vi "DB UI - MasterData SAPProduction Long Text.vi"(7 "DB Connection":T3={"Open"=TRUE, "Close"=TRUE}, 8 "error in (no error)":errorcluster, 9 "[OrderNo]":string, 10 "[PlantId]":string, 11 "connection reference 2":T1) -> (0 "SUMMARY":errorcluster, 3 "connection reference":T1)   [LabVIEW 2013]
uses:
  <vilib>/addons/database/Connection.llb/Conn ObjectReference.ctl
  Controls/DB - OpenClose.ctl
  <vilib>/Utility/miscctls.llb/LVPointTypeDef.ctl
  Controls/Global SRTRS.vi
  <vilib>/addons/database/Connection.llb/DB Tools Open Connec (String).vi
  <vilib>/addons/database/NI_Database_API.lvlib
panel:
  in  "Tab Control":enum32{"Debug"}(tab)
  out "Connection Information":T2={"Connection "="SQL Server 32bit HPEnvy", "Username"="admin", "Password"="admin123"}
  in  "SRTRS.MasterData.SAPProduction":string="SRTRS.MasterData.SAPProduction"
  out "SQL Statement":string
  out "Close 2":errorcluster
  out "[LongText]":string caption="Long Text"
  in  "Close":bool caption="Setup Save"
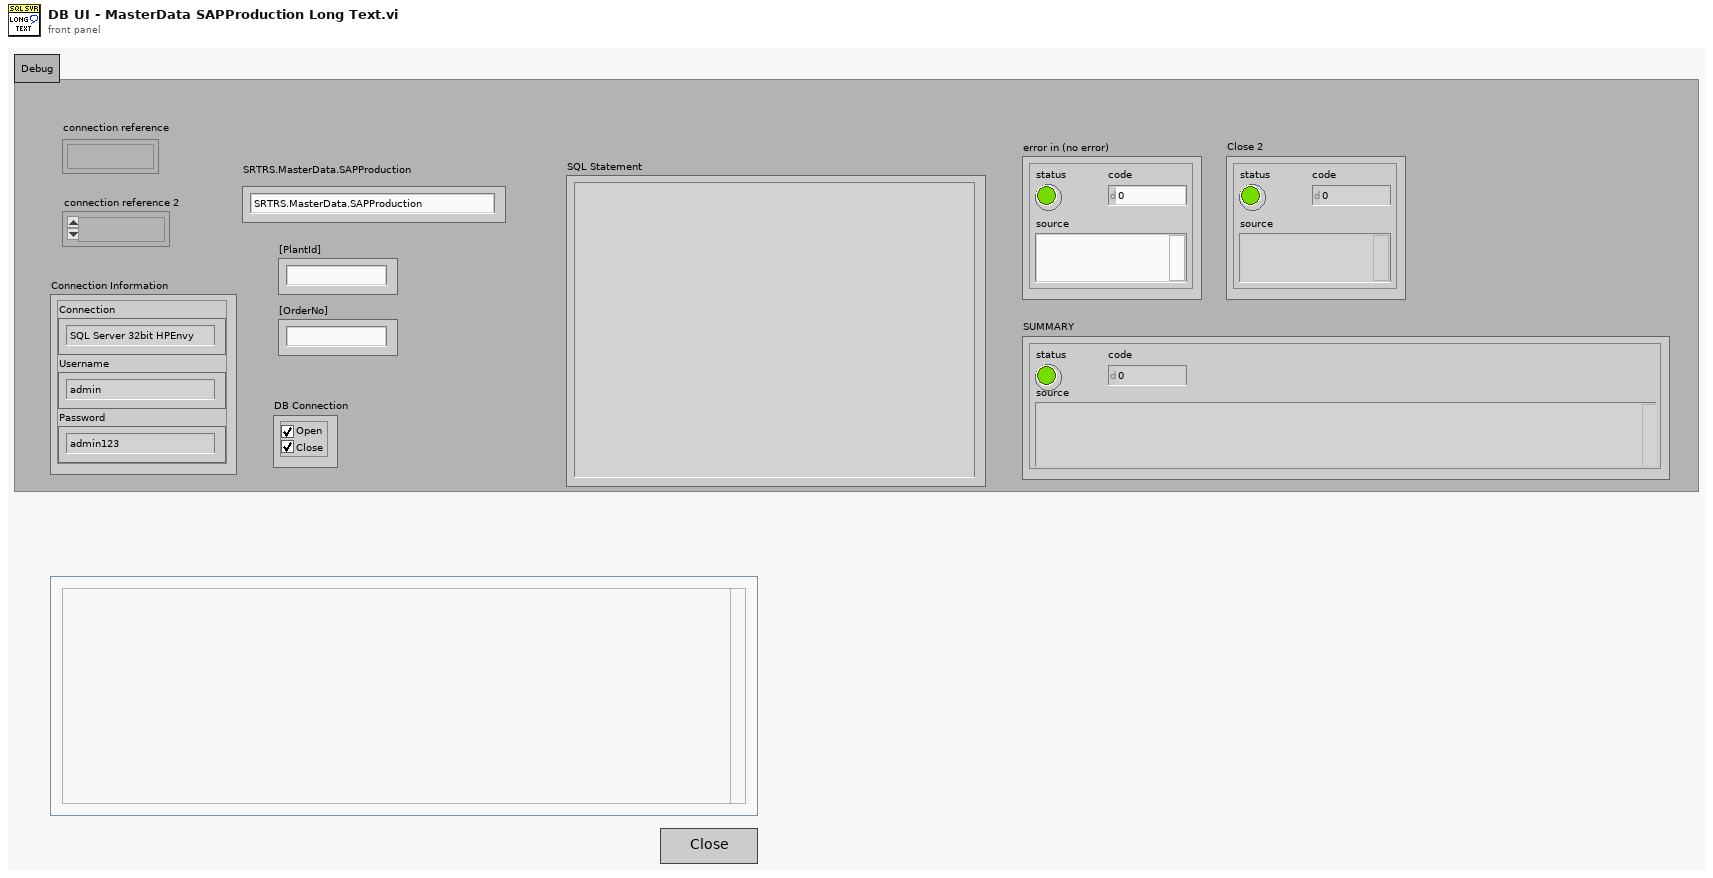
[diagram p1: front panel]
types:
  T1 = typedef "NI_Database_API.lvlib/Conn ObjectReference.ctl" = refnum<k1>
  T2 = cluster{"Connection ":string, "Username":string, "Password":string}
  T3 = typedef "DB - OpenClose.ctl" = cluster{"Open":bool, "Close":bool}
  T4 = typedef "LVPointTypeDef.ctl" = cluster{"Horizontal":i16, "Vertical":i16}
  T5 = typedef "Enum - InteractiveMode-SubVIMode.ctl" = enum16{"Interactive", "subVI Mode"}
  T6 = typedef "DB - DB.Schema.Table.ctl" = cluster{"DB":string, "Schema":string, "Table":string}
  T7 = typedef "Connection Information Cluster.ctl" = cluster{"Connection ":string, "Username":string, "Password":string}
  T8 = typedef "DB - Logon Extra Info.ctl" = cluster{"Plant Name":string, "UserName":string, "Hostname [ClientName]":string, "IsUnicode":bool}
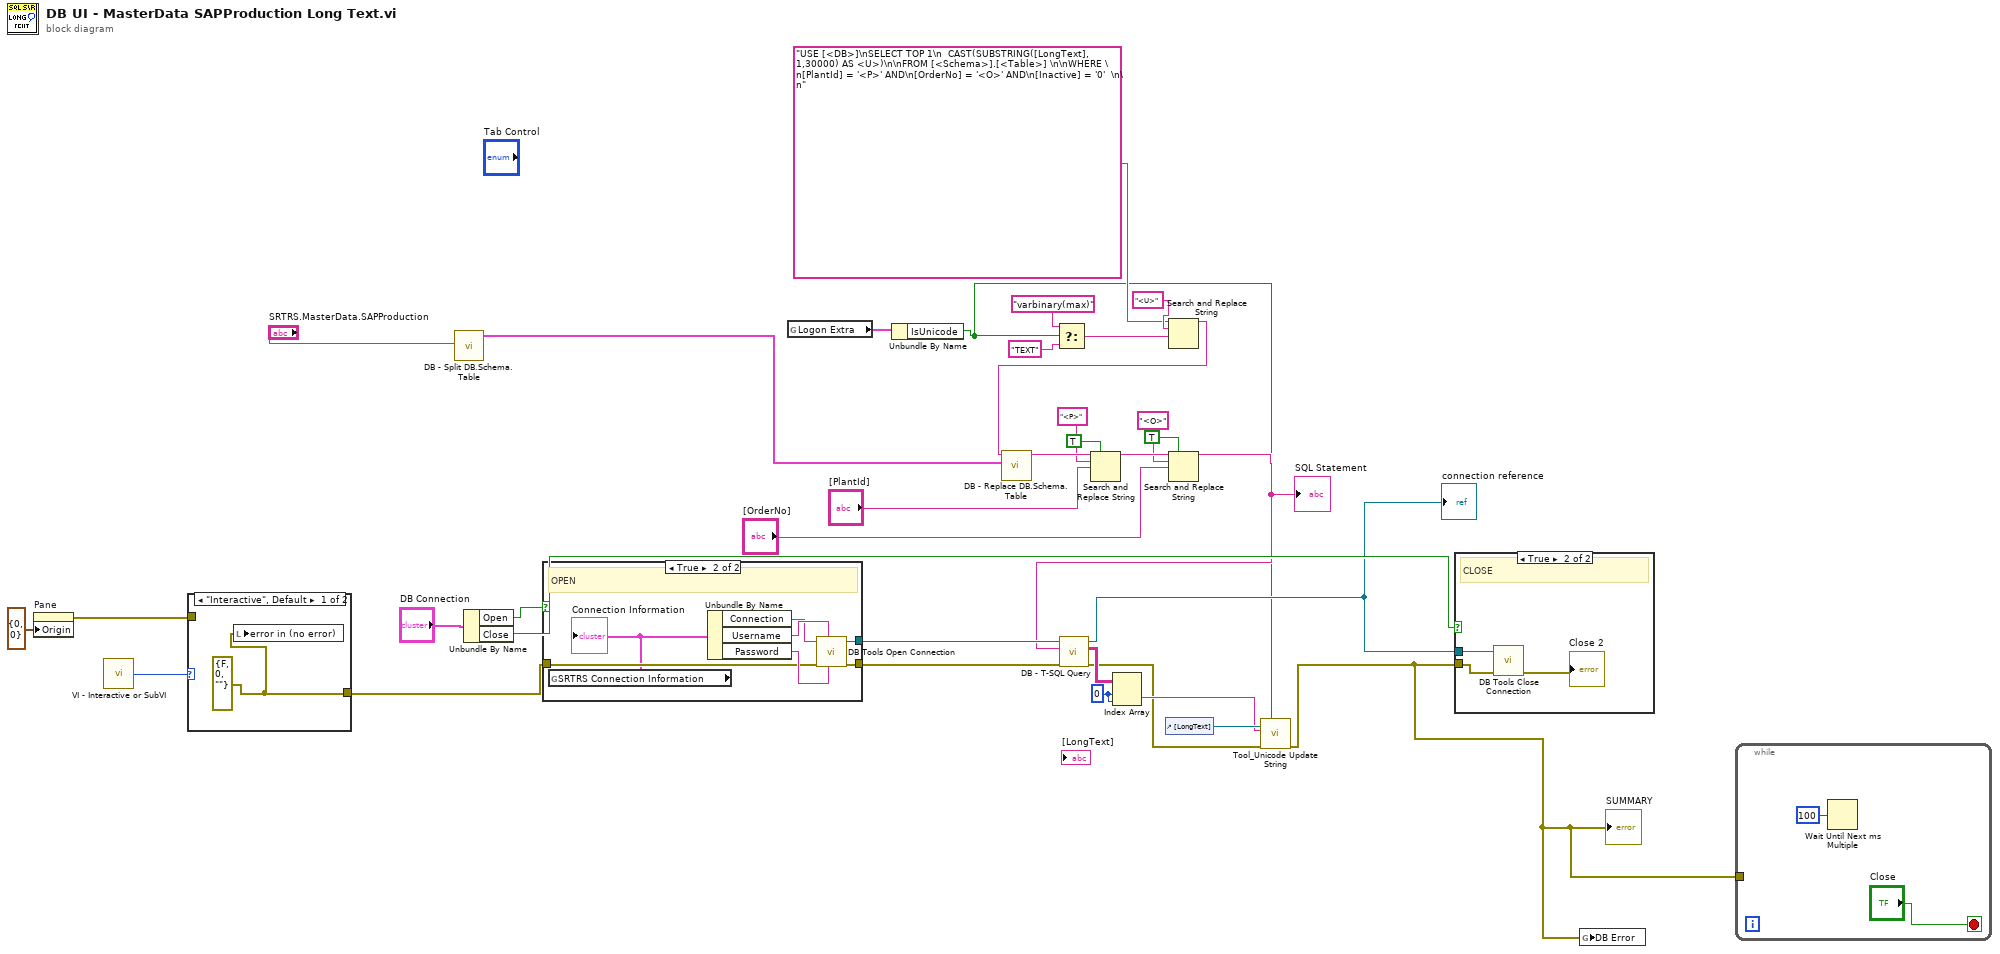
[diagram p0: block diagram]
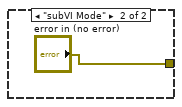
[diagram p3: hidden frame]
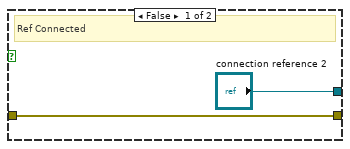
[diagram p4: hidden frame]
diagram:
  w20 = 0 ("index (row)")
  n1 = property on="Pane" class="Pane"("Origin"=T4 {"Horizontal"=0, "Vertical"=0}) -> (error out=w24:errorcluster)  [unwired: 2 in, 1 out]
  n2 = call "VI - Interactive or SubVI.vi"() -> ("Mode"=w33:T5)  [unwired: 5 in]
  n3 = case shown="\"Interactive\", Default" w33 {
    tunnel: [w36 "error in (no error)"] -> w32
    tunnel: w24 -> [_ _]
    frame "Interactive", Default {
      w36 = errorcluster {"status"=FALSE, "code"=0, "source"=""} ("error in (no error)")
      n4 = local write "error in (no error)"(w36) -> ()
    }
    frame "subVI Mode" {
    }
  }
  n5 = call "DB - Split DB.Schema.Table.vi"("DB.Schema.Table"="SRTRS.MasterData.SAPProduction") -> ("DB.Schema.Table"=w29:T6)  [unwired: 10 in]
  n6 = Unbundle By Name("DB Connection") -> ("Open"=w34:bool, "Close"=w31:bool)
  n7 = case shown="True" w34 {
    tunnel: ["connection reference 2" w43] -> w23
    tunnel: w32 -> [w38 w42]
    tunnel: [w38 w41] -> w22
    frame False {
      # "Ref Connected"
    }
    frame True {
      # "OPEN"
      n8 = global read "Global SRTRS.vi" "SRTRS Connection Information"() -> (w40:T7)
      "Connection Information" <- w40
      n9 = Unbundle By Name(w40) -> ("Connection"=w45:string, "Username"=w46:string, "Password"=w44:string)
      n10 = call-poly <vilib>:"DB Tools Open Connection.vi"("password"=w44, "userID"=w46, "error in (no error)"=w42, "connection information"=w45) -> ("error out"=w41:errorcluster, "connection reference"=w43:T1)  [unwired: 4 in]
    }
  }
  n11 = global read "Global SRTRS.vi" "Logon Extra"() -> (w6:T8)
  n12 = Unbundle By Name(w6) -> ("IsUnicode"=w5:bool)
  n13 = Select(t="varbinary(max)", s=w5, f="TEXT") -> (s? t:f=w11:string)
  n14 = control-ref of="[LongText]"() -> (w4:refnum<vi>)
  n15 = Search and Replace String(input string="USE [<DB>]\nSELECT TOP 1\n  CAST(SUBSTRING([LongText], 1,30000) AS <U>)\n\nFROM [<Schema>].[<Table>] \n\nWHERE \n[PlantId] = '<P>' AND\n[OrderNo] = '<O>' AND\n[Inactive] = '0'  \n\n", search string="<U>", replace string=w11) -> (result string=w7:string)  [unwired: 5 in, 3 out]
  n16 = call "DB - Replace DB.Schema.Table.vi"("DB.Schema.Table"=w29, "string in"=w7) -> ("string out"=w28:string)  [unwired: 8 in, 1 out]
  n17 = Search and Replace String(replace all?=TRUE ("replace all? (F)"), input string=w28, search string="<P>", replace string="[PlantId]") -> (result string=w18:string)  [unwired: 4 in, 3 out]
  n18 = Search and Replace String(replace all?=TRUE ("replace all? (F)"), input string=w18, search string="<O>", replace string="[OrderNo]") -> (result string=w17:string)  [unwired: 4 in, 3 out]
  "SQL Statement" <- w17
  n19 = call "DB - T-SQL Query.vi"("error in (no error)"=w22, "T-SQL"=w17, "connection reference"=w23) -> ("error out"=w2:errorcluster, "2D data"=w21:string[][], "connection reference"=w13:T1)  [unwired: 6 in]
  "connection reference" <- w13
  n20 = Index Array(array=w21, index (row)=w20, index (col)=w20) -> (element=w3:string)
  n21 = call "Tool_Unicode Update String.vi"("Interpret as Unicode (T)"=w5, "error in (no error)"=w2, "String Value"=w3, "String Control Reference"=w4) -> ("error out"=w1:errorcluster)  [unwired: 4 in, 1 out]
  "SUMMARY" <- w1
  n22 = case shown="True" w31 {
    tunnel: w13 -> [_ w49]
    tunnel: w1 -> [_ w48]
    frame False {
      # "Ref Connected"
    }
    frame True {
      # "CLOSE"
      n23 = call <vilib>:"DB Tools Close Connection.vi"("error in (no error)"=w48, "connection reference"=w49) -> ("error out"=→"Close 2":errorcluster)  [unwired: 5 in]
    }
  }
  n24 = global write "Global SRTRS.vi" "DB Error"(w1) -> ()
  n25 = while {
    tunnel: w1 -> [_]
    stop <- "Close" stop-if-true
    n26 = Wait Until Next ms Multiple(millisecond multiple=u32 100) -> ()  [unwired: 1 out]
  }
